vi "LauncherFeeder.vi"(2 "Target RPM F":dbl=770.0, 3 "Target RPM":dbl=3300.0) -> (0 "RPM F":dbl=3319.8279051826034, 1 "RPM L":dbl=3319.8279051826034)   [LabVIEW 2016]
doc: "This example shows how to move a motor connected to an encoder and a wheel, and then read information about the system from an encoder.\n\nThis is an example of how to use feedback (from the encoder) to create an open loop system. If some control method was used, for example using PID, a closed loop system could be created.\n\nThis example expects a USB cable connected from your development PC to the Type B USB Jack (next to the power input) on the roboRIO.\n\nThis example requires the Driver Station to be running with Teleoperated Enabled."
uses:
  <vilib>/gmath/NI_Gmath.lvlib
panel:
  in  "Feeder Enabled":bool=TRUE
  out "DS Original F":dbl=0.6428571428571428
  in  "Lower Limit F":dbl=-50.0 format="%#_13g"
  in  "Upper Limit F":dbl=50.0 format="%#_13g"
  in  "Pos Drive Signal F":dbl=0.4
  in  "Neg Drive Signal F":dbl=0.05
  out "Error F":dbl=-19.827905182603445
  out "Encoder Alarm Status F":string="Encoder Moving"
  out "Encoder Direction F":string="Forward"
  in  "Lower Limit L":dbl=-50.0 format="%#_13g"
  in  "Upper Limit L":dbl=50.0 format="%#_13g"
  out "Error L":dbl=-19.827905182603445
  out "DS Original L":dbl=0.6428571428571428
  in  "Neg Drive Signal":dbl=0.6
  in  "Pos Drive Signal":dbl=1.0
  in  "MS to Wait":u32=10
  out "Loop Time (s)":dbl=0.010378 format="%_6f"
  out "Encoder Alarm Status L":string="Encoder Moving"
  out "Encoder Direction L":string="Forward"
  # "These can be set while running."
  # "Output information."
  # "Need to tune target RPM and drive signals"
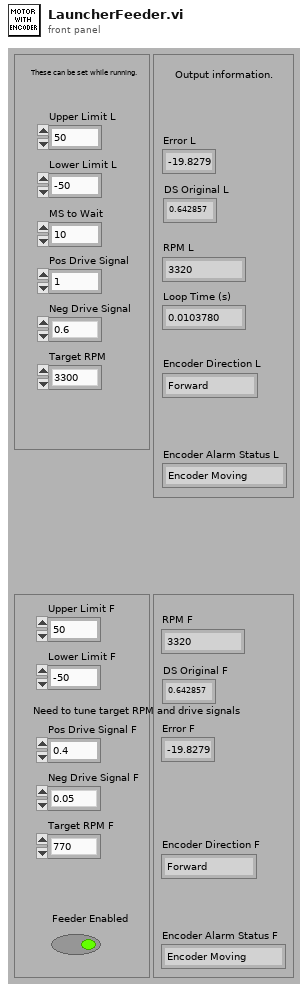
[diagram p1: front panel]
types:
  T1 = typedef "WPI_EncoderDevRef.ctl" = cluster{"DevStatus":errorcluster, "EncoderIndex":T2, "CounterIndex":T3, "DistancePerCount":dbl, "Decoding Type":T4}
  T2 = typedef "FPGA_EncoderIdx.ctl" = enum8{"Enc 0", "Enc 1", "Enc 2", "Enc 3", "Enc 4", "Enc 5", "Enc 6", "Enc 7", "Invalid"}
  T3 = typedef "FPGA_CounterCtrSystemIndex.ctl" = enum8{"Ctr 0", "Ctr 1", "Ctr 2", "Ctr 3", "Ctr 4", "Ctr 5", "Ctr 6", "Ctr 7", "Invalid"}
  T4 = typedef "WPI_EncoderType.ctl" = enum16{"1x", "2x", "4x"}
  T5 = typedef "WPI_MotorControlDeviceRef.ctl" = cluster{"DeviceStatus":errorcluster, "Type":T6, "PWM":cluster{"PWM Channel":T7, "DeadBand":T8}, "CAN":cluster{"Device Number":u8, "SetOutput VI Ref":variant, "GetOutput VI Ref":variant, "Enable VI Ref":variant, "Disable VI Ref":variant, "Data":variant}, "Invert":bool}
  T6 = typedef "WPI_MotorControlType.ctl" = enum16{"PWM", "CAN"}
  T7 = typedef "FPGA_DIOPWMChannel.ctl" = enum8{"PWM 0", "PWM 1", "PWM 2", "PWM 3", "PWM 4", "PWM 5", "PWM 6", "PWM 7", "PWM 8", "PWM 9", "PWM MXP 0", "PWM MXP 1", "PWM MXP 2", "PWM MXP 3", "PWM MXP 4", "PWM MXP 5", "PWM MXP 6", "PWM MXP 7", "PWM MXP 8", "PWM MXP 9", "Invalid"}
  T8 = typedef "WPI_PWMDeadband.ctl" = cluster{"Name":string, "maxPositivePwm":i32, "minPositivePwm":i32, "centerPwm":i32, "maxNegativePwm":i32, "minNegativePwm":i32, "angularRange":u16}
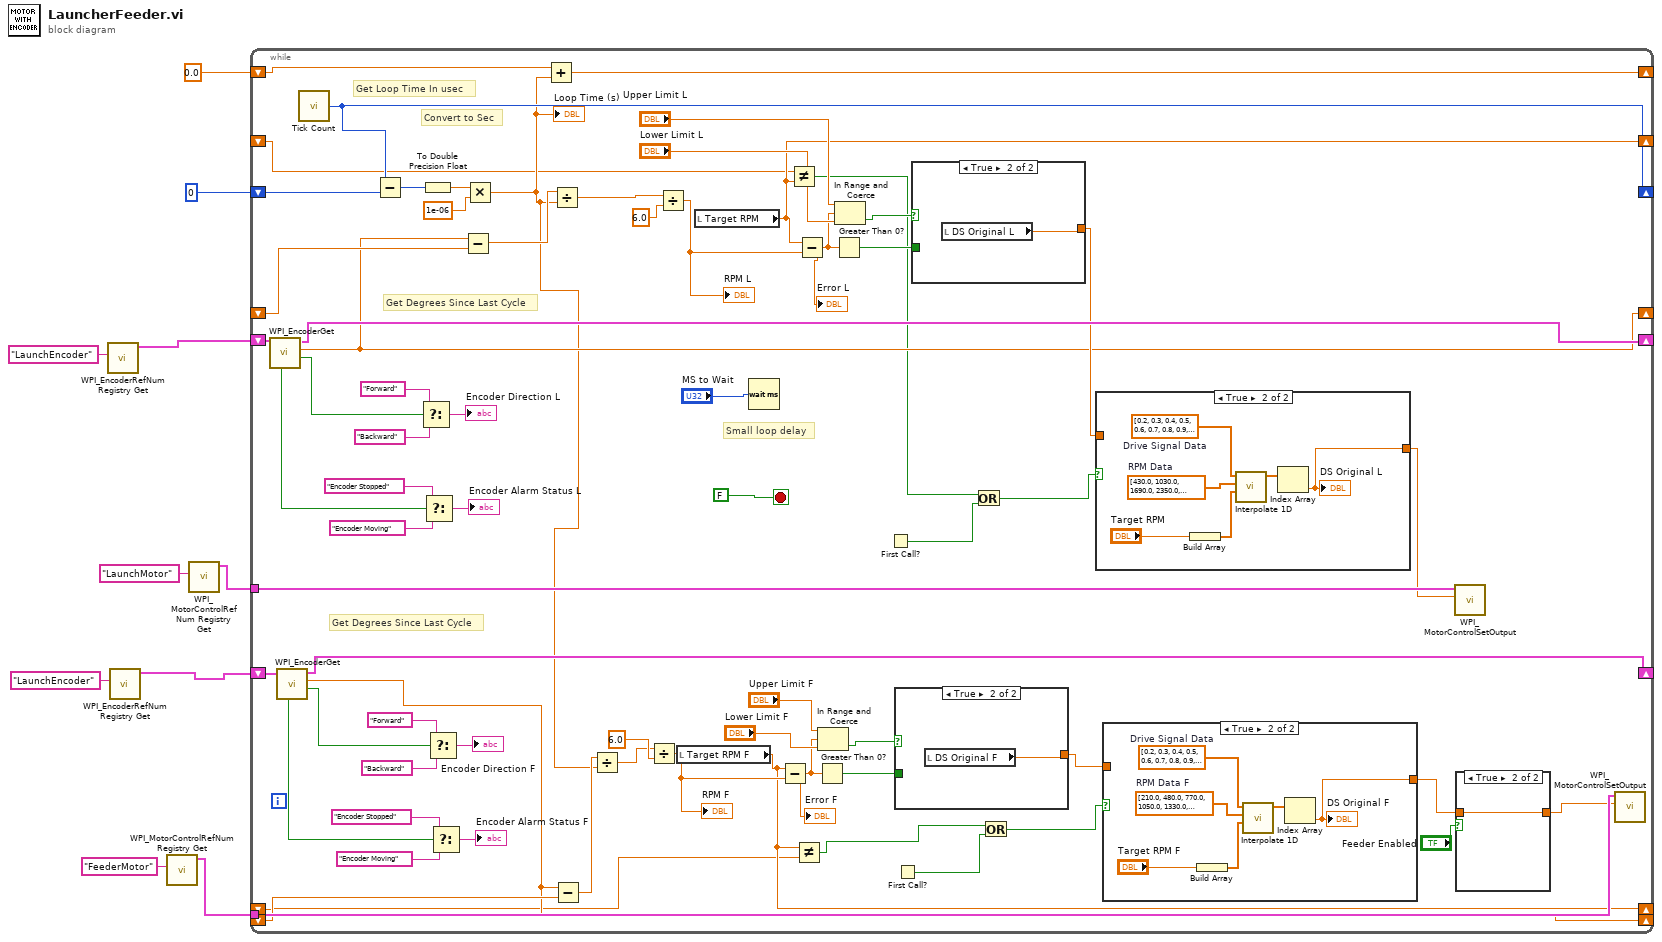
[diagram p0: block diagram]
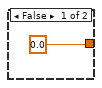
[diagram p2: hidden frame]
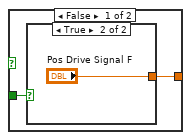
[diagram p4: hidden frame]
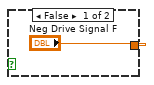
[diagram p5: hidden frame]
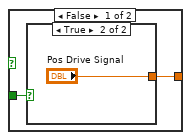
[diagram p7: hidden frame]
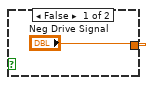
[diagram p8: hidden frame]
diagram:
  n1 = call <vilib>:"WPI_EncoderRefNum Registry Get.vi"("refnum name"="LaunchEncoder") -> ("EncoderDevRef"=w1:T1)  [unwired: 9 in, 1 out]
  n2 = call <vilib>:"WPI_EncoderRefNum Registry Get.vi"("refnum name"="LaunchEncoder") -> ("EncoderDevRef"=w2:T1)  [unwired: 9 in, 1 out]
  n3 = call <vilib>:"WPI_MotorControlRefNum Registry Get.vi"("refnum name"="FeederMotor") -> ("MotorControlDevRef"=w5:T5)  [unwired: 9 in, 1 out]
  n4 = call <vilib>:"WPI_MotorControlRefNum Registry Get.vi"("refnum name"="LaunchMotor") -> ("MotorControlDevRef"=w7:T5)  [unwired: 9 in, 1 out]
  n5 = while {
    shift-right: [w67] -> _
    shift-left: w1 -> [w70]
    tunnel: w7 -> [w72]
    shift-right: [w66] -> _
    shift-left: u32 0 ("Tick Count(uSec)") -> [w65]
    shift-right: [w46] -> _
    shift-left: _ -> [w64]
    shift-right: [w57] -> _
    shift-left: 0.0 ("Tick Count(uSec)") -> [w58]
    tunnel: w5 -> [w26]
    shift-right: [w24] -> _
    shift-left: w2 -> [w25]
    shift-right: [w18] -> _
    shift-left: _ -> [w22]
    shift-right: [w16] -> _
    shift-left: _ -> [w15]
    shift-right: [w13] -> _
    shift-left: _ -> [w12]
    stop <- FALSE ("Stop") stop-if-true
    # "Get Degrees Since Last Cycle"
    # "Get Degrees Since Last Cycle"
    # "Convert to Sec"
    # "Get Loop Time In usec"
    # "Small loop delay"
    n6 = call <vilib>:"WPI_EncoderGet.vi"("EncoderDevRef"=w70) -> ("Direction"=w78:bool, "Distance"=w46:dbl, "EncoderDevRef"=w67:T1, "Stopped"=w77:bool)  [unwired: 1 in, 6 out]
    n7 = call <vilib>:"WPI_EncoderGet.vi"("EncoderDevRef"=w25) -> ("Direction"=w43:bool, "Distance"=w18:dbl, "EncoderDevRef"=w24:T1, "Stopped"=w42:bool)  [unwired: 1 in, 6 out]
    n8 = call "Tick Count"() -> ("Tick Count(uSec)"=w66:u32)
    n9 = Subtract(x=w66, y=w65) -> (x-y=w63:u32)
    n10 = Select(t="Forward", s=w78, f="Backward") -> (s? t:f=→"Encoder Direction L":string)
    n11 = To Double Precision Float(number=w63) -> (double precision float=w61:dbl)
    n12 = Select(t="Encoder Stopped", s=w77, f="Encoder Moving") -> (s? t:f=→"Encoder Alarm Status L":string)
    n13 = Select(t="Forward", s=w43, f="Backward") -> (s? t:f=→"Encoder Direction F":string)
    n14 = Select(t="Encoder Stopped", s=w42, f="Encoder Moving") -> (s? t:f=→"Encoder Alarm Status F":string)
    n15 = Subtract(x=w46, y=w64) -> (x-y=w60:dbl)
    n16 = Multiply(x=w61, y=1e-06) -> (x*y=w17:dbl)
    "Loop Time (s)" <- w17
    n17 = Add(x=w58, y=w17) -> (x+y=w57:dbl)
    n18 = Divide(x=w60, y=w17) -> (x/y=w59:dbl)
    n19 = Subtract(x=w18, y=w22) -> (x-y=w36:dbl)
    n20 = Divide(x=w36, y=w17) -> (x/y=w35:dbl)
    n21 = Divide(x=w35, y=6.0) -> (x/y=w27:dbl)
    "RPM F" <- w27
    n22 = Divide(x=w59, y=6.0) -> (x/y=w56:dbl)
    "RPM L" <- w56
    n23 = local read "Target RPM F"() -> (w13:dbl)
    n24 = local read "Target RPM"() -> (w16:dbl)
    n25 = Wait (ms)(milliseconds to wait="MS to Wait") -> ()  [unwired: 1 out]
    n26 = Subtract(x=w13, y=w27) -> (x-y=w30:dbl)
    "Error F" <- w30
    n27 = Not Equal?(x=w15, y=w16) -> (x != y?=w14:bool)
    n28 = Not Equal?(x=w13, y=w12) -> (x != y?=w11:bool)
    n29 = Subtract(x=w16, y=w56) -> (x-y=w51:dbl)
    "Error L" <- w51
    n30 = Greater Than 0?(x=w30) -> (x > 0?=w34:bool)
    n31 = In Range and Coerce(upper limit="Upper Limit F", x=w30, lower limit="Lower Limit F") -> (In Range?=w31:bool)  [unwired: 1 out]
    n32 = Greater Than 0?(x=w51) -> (x > 0?=w55:bool)
    n33 = In Range and Coerce(upper limit="Upper Limit L", x=w51, lower limit="Lower Limit L") -> (In Range?=w52:bool)  [unwired: 1 out]
    n34 = First Call?() -> (First Call?: T/F=w47:bool)
    n35 = First Call?() -> (First Call?: T/F=w28:bool)
    n36 = case shown="True" w31 {
      tunnel: w34 -> [w91 _]
      tunnel: [w90 w94] -> w23
      frame False {
        n37 = case shown="True" w91 {
          tunnel: ["Neg Drive Signal F" "Pos Drive Signal F"] -> w90
          frame False {
          }
          frame True {
          }
        }
      }
      frame True {
        n38 = local read "DS Original F"() -> (w94:dbl)
      }
    }
    n39 = case shown="True" w52 {
      tunnel: w55 -> [w103 _]
      tunnel: [w102 w106] -> w50
      frame False {
        n40 = case shown="True" w103 {
          tunnel: ["Neg Drive Signal" "Pos Drive Signal"] -> w102
          frame False {
          }
          frame True {
          }
        }
      }
      frame True {
        n41 = local read "DS Original L"() -> (w106:dbl)
      }
    }
    n42 = Or(x=w14, y=w47) -> (x .or. y?=w48:bool)
    n43 = Or(x=w11, y=w28) -> (x .or. y?=w29:bool)
    n44 = case shown="True" w48 {
      tunnel: [w95 w96] -> w49
      tunnel: w50 -> [w95 _]
      frame False {
      }
      frame True {
        w101 = dbl[] [430.0, 1030.0, 1690.0, 2350.0, 3000.0, 3700.0, 4400.0, 5000.0, 5550.0]  # RPM Data
        w100 = dbl[] [0.2, 0.3, 0.4, 0.5, 0.6, 0.7, 0.8, 0.9, 1.0]  # Drive Signal Data
        n45 = Build Array("Target RPM") -> (w98:dbl[])
        n46 = call <vilib>:"Interpolate 1D.vi"("xi"=w98, "X"=w101, "Y"=w100) -> ("yi"=w97:dbl[])  [unwired: 6 in, 2 out]
        n47 = Index Array(array=w97) -> (element=w96:dbl)  [unwired: 1 in]
        "DS Original L" <- w96
      }
    }
    n48 = case shown="True" w29 {
      tunnel: [w83 w84] -> w21
      tunnel: w23 -> [w83 _]
      frame False {
      }
      frame True {
        w89 = dbl[] [210.0, 480.0, 770.0, 1050.0, 1330.0, 1650.0, 1870.0, 2140.0, 2400.0]  # RPM Data F
        w88 = dbl[] [0.2, 0.3, 0.4, 0.5, 0.6, 0.7, 0.8, 0.9, 1.0]  # Drive Signal Data
        n49 = Build Array("Target RPM F") -> (w86:dbl[])
        n50 = call <vilib>:"Interpolate 1D.vi"("xi"=w86, "X"=w89, "Y"=w88) -> ("yi"=w85:dbl[])  [unwired: 6 in, 2 out]
        n51 = Index Array(array=w85) -> (element=w84:dbl)  [unwired: 1 in]
        "DS Original F" <- w84
      }
    }
    n52 = call <vilib>:"WPI_MotorControlSetOutput.vi"("Output"=w49, "MotorControlDevRef"=w72) -> ()  [unwired: 2 in, 8 out]
    n53 = case shown="True" "Feeder Enabled" {
      tunnel: [0.0 w82] -> w20
      tunnel: w21 -> [_ w82]
      frame False {
      }
      frame True {
      }
    }
    n54 = call <vilib>:"WPI_MotorControlSetOutput.vi"("Output"=w20, "MotorControlDevRef"=w26) -> ()  [unwired: 2 in, 8 out]
  }
